vi "Write Remote IP Address.vi"(10 "Remote IP":string, 11 "TCP Stream in":refnum<class "TCP Stream.lvclass">) -> (3 "TCP Stream out":refnum<class "TCP Stream.lvclass">)   [LabVIEW 2020, in "TCP Stream.lvclass"]
doc: "Use this VI to specify the remote IP address to use for this connection."
uses:
  TCP Stream.lvclass
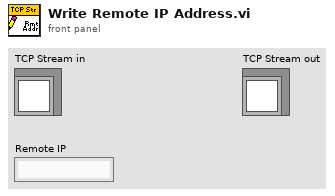
[diagram p1: front panel]
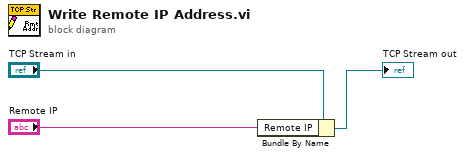
[diagram p0: block diagram]
diagram:
  n1 = Bundle By Name(cluster="TCP Stream in", "Remote IP"="Remote IP") -> (→"TCP Stream out":refnum<class "TCP Stream.lvclass">)
